vi "LabJackU6_Read_New.vi"(8 "error in":errorcluster, 10 "n_samples":i32=10, 11 "Handle In":i32) -> (0 "error out":errorcluster, 1 "AI2":dbl, 2 "AI0":dbl, 3 "Handle Out":i32)   [LabVIEW 2019]
uses:
  <vilib>/Analysis/baseanly.llb/Mean (DBL).vi
  <vilib>/Analysis/NI_AALBase.lvlib
panel:
  out "Values Read":dbl[][](array[numeric])
  out "Mean array":dbl[](array[numeric])
  in  "Channels":i32[](array[numeric])
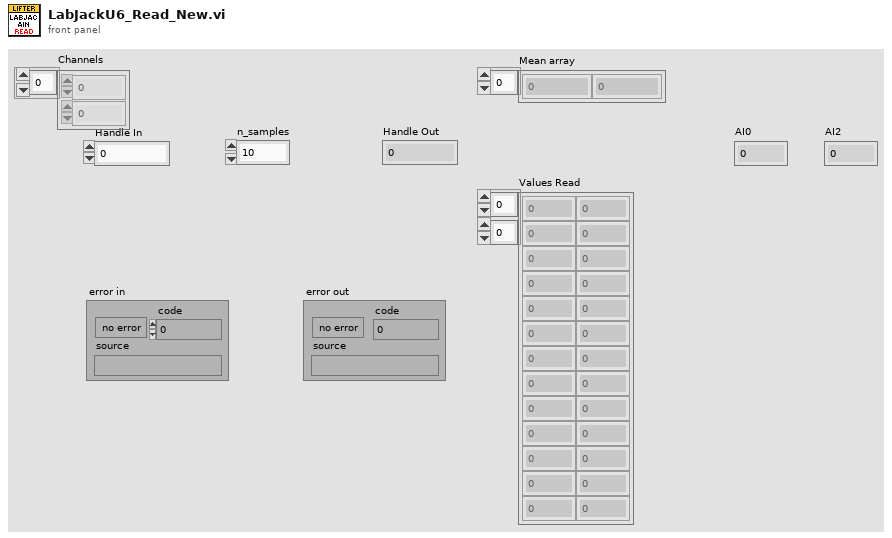
[diagram p1: front panel]
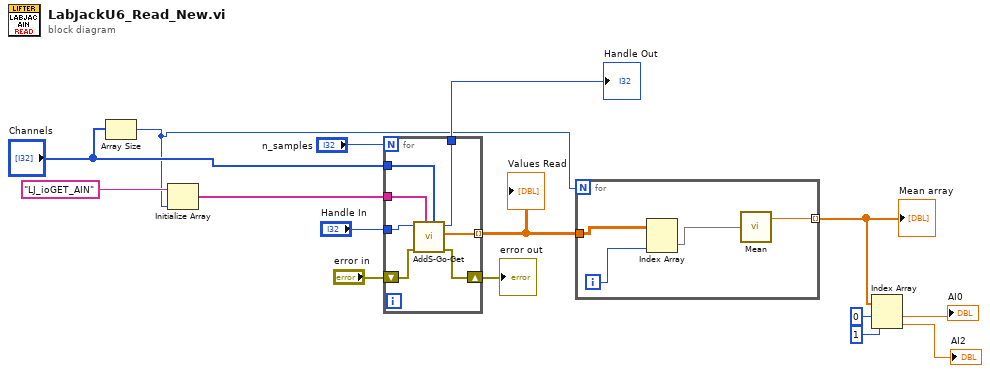
[diagram p0: block diagram]
diagram:
  n1 = Array Size(array="Channels") -> (size(s)=w6:i32)
  n2 = Initialize Array("LJ_ioGET_AIN", w6) -> (w10:string[])
  n3 = for {
    N: "n_samples" -> [_]
    shift-right: [w16] -> w13
    shift-left: "error in" -> [w17]
    tunnel: "Handle In" -> [w18]
    tunnel: w10 -> [w22]
    tunnel: "Channels" -> [w21]
    tunnel: [w20] -> w8
    tunnel: [w19] -> w7 mode=indexing
    n4 = call "AddS-Go-Get.vi"("Channels"=w21, "IOTypes"=w22, "error in"=w17, "Handle In"=w18) -> ("error out"=w16:errorcluster, "Values Read"=w19:dbl[], "Handle Out"=w20:i32)  [unwired: 5 in]
  }
  "error out" <- w13
  "Handle Out" <- w8
  "Values Read" <- w7
  n5 = for {
    N: w6 -> [_]
    tunnel: [w26] -> w1 mode=indexing
    tunnel: w7 -> [w25]
    i -> [w24]
    n6 = Index Array(array=w25, index (col)=w24) -> (element=w23:dbl[])  [unwired: 1 in]
    n7 = call-poly <vilib>:"Mean.vi"("X"=w23) -> ("mean"=w26:dbl)  [unwired: 1 out]
  }
  "Mean array" <- w1
  n8 = Index Array(array=w1, index #1=0 ("index"), index #2=1 ("index")) -> (element #1=→"AI0":dbl, element #2=→"AI2":dbl)
